vi "Socket Opened.vi"(8 "error in":errorcluster) -> (0 "error out":errorcluster)   [LabVIEW 2019, in "RemoteControl.ZMQ.lvlib" / "ZMQ.ContextManager.lvlib"]
uses:
  ZMQ.ContextManager.lvlib
  Typedefs/Action--enum.ctl
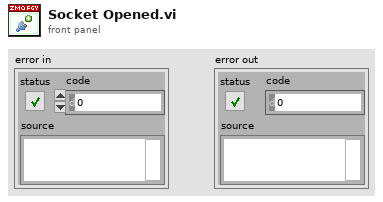
[diagram p1: front panel]
types:
  T1 = typedef "RemoteControl.ZMQ.lvlib/ZMQ.ContextManager.lvlib/Action--enum.ctl" = enum16{"Get Context", "Release Context", "Socket Opened", "Socket Closed", "Force Cleanup"}
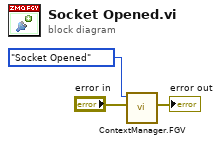
[diagram p0: block diagram]
diagram:
  n1 = call "ContextManager.FGV.vi"("error in"="error in", "action"=Action--enum."Socket Opened") -> ("error out"=→"error out":errorcluster)  [unwired: 8 in, 1 out]
